vi "makeCurrentMonth.vi"(8 "error in (no error)":errorcluster, 11 "MonthDisplay in":refnum<class "DateUserInterface.lvclass">) -> (0 "error out":errorcluster, 3 "MonthDisplay out":refnum<class "DateUserInterface.lvclass">)   [LabVIEW 2020, in "DateUserInterface.lvclass"]
uses:
  DateUserInterface.lvclass
  month.ctl
  DateUserInterface.lvclass/DateUserInterface.ctl
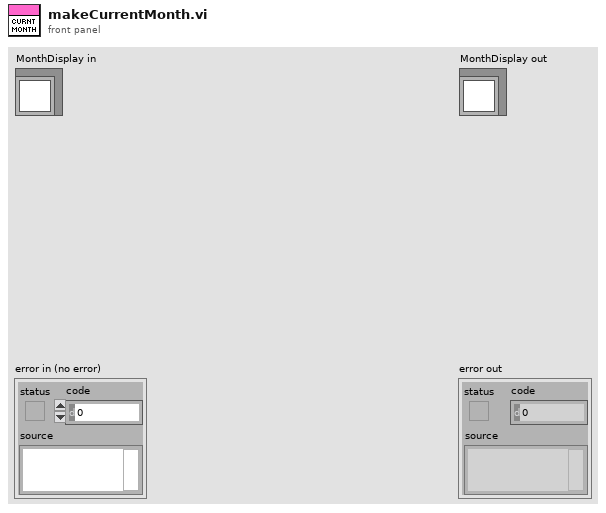
[diagram p1: front panel]
types:
  T1 = typedef "DateUserInterface.lvclass/month.ctl" = enum16{"January", "February", "March", "April", "May", "June", "July", "August", "September", "October", "November", "December"}
  T2 = typedef "LVDateTimeRec.ctl" = cluster{"fractional second":dbl, "second":i32, "minute":i32, "hour":i32, "day of month":i32, "month":i32, "year":i32, "day of week":i32, "day of year":i32, "DST":i32}
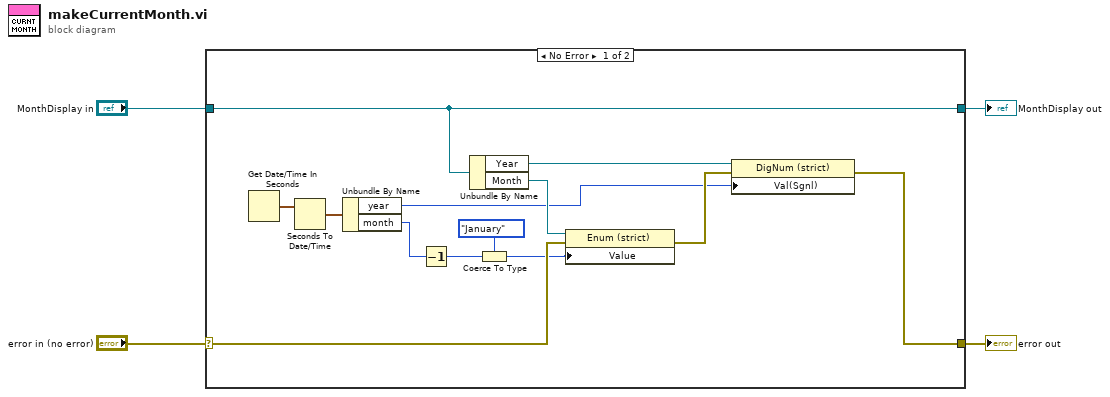
[diagram p0: block diagram]
diagram:
  n1 = case shown="No Error" "error in (no error)" {
    selector: "error in (no error)" -> [w15 w19]
    tunnel: [w13 w19] -> w3
    tunnel: [w17 w18] -> w1
    tunnel: "MonthDisplay in" -> [w17 w18]
    frame No Error {
      n2 = Get Date/Time In Seconds() -> (seconds since 1Jan1904=w7:timestamp)
      n3 = Seconds To Date/Time(time stamp (now)=w7) -> (date time rec=w8:T2)  [unwired: 1 in]
      n4 = Unbundle By Name(w8) -> ("year"=w6:i32, "month"=w5:i32)
      n5 = Decrement(x=w5) -> (x-1=w12:i32)
      n6 = Unbundle By Name(w17) -> ("Year"=w16:refnum<vi>, "Month"=w9:refnum<vi>)
      n7 = Coerce To Type(0:w12, 1:month."January" ("Month")) -> (2:w10:T1)
      n8 = property class="Enum (strict)"(reference=w9, error in=w15, "Value"=w10) -> (error out=w14:errorcluster)  [unwired: 1 out]
      n9 = property class="DigNum (strict)"(reference=w16, error in=w14, "Val(Sgnl)"=w6) -> (error out=w13:errorcluster)  [unwired: 1 out]
    }
    frame Error {
    }
  }
  "error out" <- w3
  "MonthDisplay out" <- w1
